vi "Shortest Distance Absolute.vi"(10 "Set point":dbl(knob) scale=0.0..360.0, 11 "Current Angle":dbl(knob) scale=0.0..360.0) -> (3 "Degres To Travel":dbl)   [LabVIEW 2011, in "Pivot Drive.lvlib"]
uses:
  Pivot Drive.lvlib
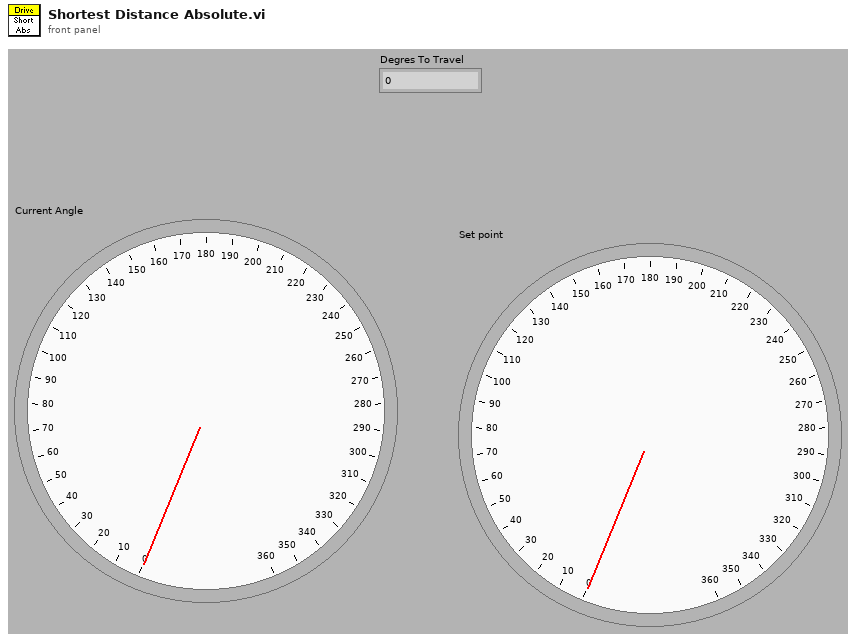
[diagram p1: front panel]
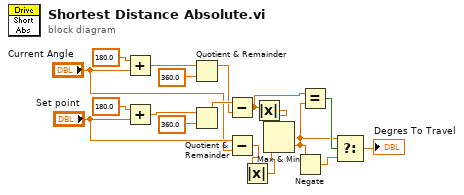
[diagram p0: block diagram]
diagram:
  n1 = Add(x=180.0, y="Current Angle") -> (x+y=w15:dbl)
  n2 = Add(x=180.0, y="Set point") -> (x+y=w12:dbl)
  n3 = Quotient & Remainder(x=w15, y=360.0) -> (x-y*floor(x/y)=w4:dbl)  [unwired: 1 out]
  n4 = Quotient & Remainder(x=w12, y=360.0) -> (x-y*floor(x/y)=w6:dbl)  [unwired: 1 out]
  n5 = Subtract(x=w6, y=w4) -> (x-y=w3:dbl)
  n6 = Subtract(x="Set point", y="Current Angle") -> (x-y=w10:dbl)
  n7 = Absolute Value(x=w10) -> (abs(x)=w9:dbl)
  n8 = Absolute Value(x=w3) -> (abs(x)=w8:dbl)
  n9 = Max & Min(x=w8, y=w9) -> (min(x,y)=w1:dbl)  [unwired: 1 out]
  n10 = Negate(x=w1) -> (-x=w2:dbl)
  n11 = Equal?(x=w3, y=w1) -> (x = y?=w17:bool)
  n12 = Select(t=w1, s=w17, f=w2) -> (s? t:f=→"Degres To Travel":dbl)
